vi "Configure Session.vi"(8 "error in":errorcluster, 11 "Plugin in":refnum<class "DateTimeChannel.lvclass">) -> (0 "error out":errorcluster, 3 "Plugin out":refnum<class "DateTimeChannel.lvclass">)   [LabVIEW 2023, in "DateTimeChannel.lvlib" / "DateTimeChannel.lvclass"]
uses:
  DateTimeChannel.lvclass
  C:/Program Files/National Instruments/LabVIEW 2023/vi.lib/FlexLogger/SDK/PluginSDK.lvlibp/PEFClasses/SDK/Plugin/Plugin.lvclass
  DateTimeChannel.lvclass/DateTimeChannel.ctl
  <vilib>/FlexLogger/SDK/PluginSDK.lvlibp/PEFClasses/SDK/Plugin/ParameterAccess/Read String.vi
  <vilib>/FlexLogger/SDK/PluginSDK.lvlibp/PEFClasses/SDK/Plugin/Plugin.lvclass
  C:/Program Files/National Instruments/LabVIEW 2023/vi.lib/FlexLogger/SDK/PluginSDK.lvlibp/PEFClasses/SDK/Processing Element/Processing Element.lvclass
  C:/Users/bbuchana/Documents/LabVIEW Projects/FlexLogger IO Plug-ins/DateTimeChannel/DateTimeChannel.lvclass
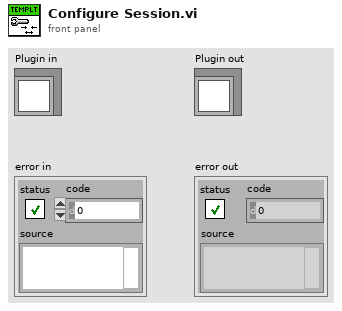
[diagram p1: front panel]
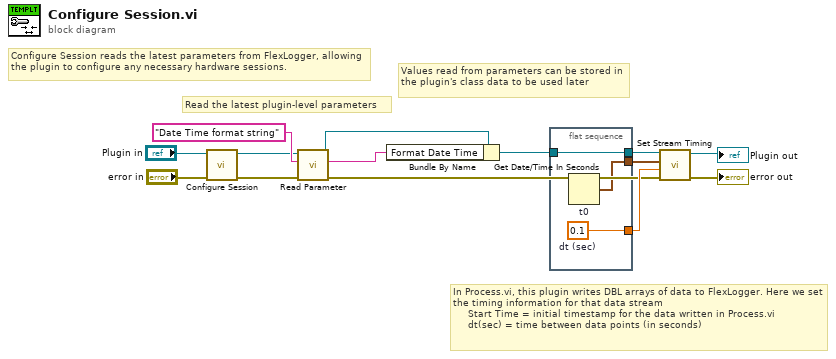
[diagram p0: block diagram]
diagram:
  # "Read the latest plugin-level parameters"
  # "Configure Session reads the latest parameters from FlexLogger, allowing the plugin to configure any necessary hardware sessions."
  # "Values read from parameters can be stored in the plugin's class data to be used later"
  # "In Process.vi, this plugin writes DBL arrays of data to FlexLogger. Here we set the timing information for that data stream\n     Start Time = initial timestamp for the data written in Process.vi\n     dt(sec) = time between data points (in seconds)"
  n1 = call-parent "Configure Session.vi"("error in (no error)"="error in", "Processing Element in"="Plugin in") -> ("error out"=w6:errorcluster, "Processing Element out"=w7:refnum<class "DateTimeChannel.lvclass">)  [unwired: 8 in]
  n2 = call-poly <vilib>:"Read Parameter.vi"("error in (no error)"=w6, "Name"="Date Time format string", "Plugin in"=w7) -> ("error out"=w3:errorcluster, "Value"=w4:string, "Plugin out"=w5:refnum<class "DateTimeChannel.lvclass">)  [unwired: 5 in, 1 out]
  n3 = Bundle By Name(cluster=w5, "Format Date Time"=w4) -> (w11:refnum<class "DateTimeChannel.lvclass">)
  n4 = flat-sequence {
    tunnel: [w17] -> w10
    tunnel: [w16] -> w9
    tunnel: w11 -> [w15]
    tunnel: [w15] -> w1
    frame #0 {
      w16 = 0.1  # dt (sec)
      n5 = Get Date/Time In Seconds "t0"() -> (seconds since 1Jan1904=w17:timestamp)
    }
  }
  n6 = call-dynamic "Set Stream Timing.vi"("error in (no error)"=w3, "dt(sec)"=w9, "Start Time"=w10, "Plugin in"=w1) -> ("error out"=→"error out":errorcluster, "Plugin out"=→"Plugin out":refnum<class "DateTimeChannel.lvclass">)  [unwired: 6 in]
